vi "JPG_Percentile.vi"(5 "max":u16=97, 7 "min":u16=3, 10 "u16 pixmap 3":T1) -> (2 "unsigned 8bit integer":u8[][](array[numeric]))   [LabVIEW 2020]
uses:
  <vilib>/gmath/NI_Gmath.lvlib
  <vilib>/gmath/statdist.llb/st_Percentiles (scalar).vi
  _controls/img.u16.graph.25pc.axes.ctl
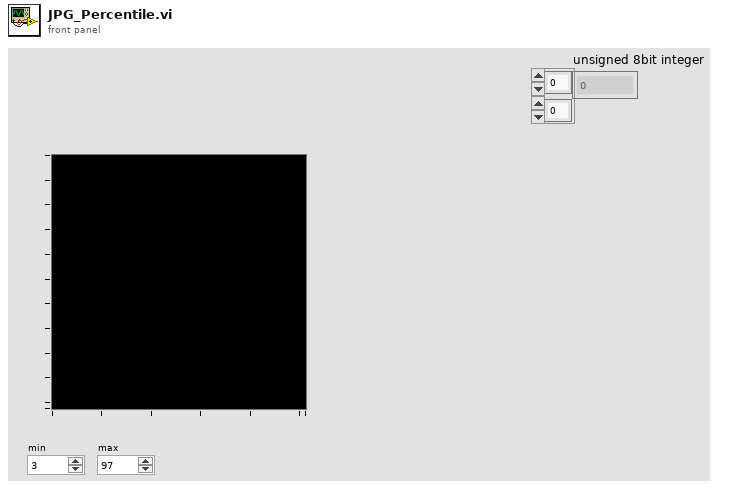
[diagram p1: front panel]
types:
  T1 = typedef "img.u16.graph.25pc.axes.ctl" = u16[][]
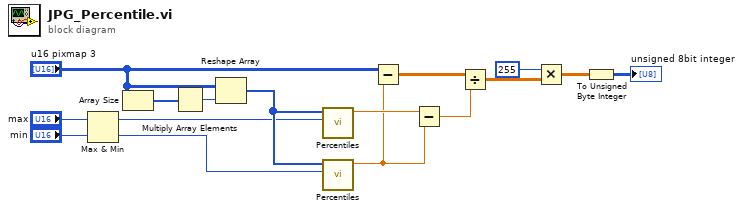
[diagram p0: block diagram]
diagram:
  n1 = Max & Min(x="max", y="min") -> (max(x,y)=w6:u16, min(x,y)=w5:u16)
  n2 = Array Size(array="u16 pixmap 3") -> (size(s)=w13:i32[])
  n3 = Multiply Array Elements(1:w13) -> (0:w12:i32)
  n4 = Reshape Array("u16 pixmap 3", w12) -> (w11:u16[])
  n5 = call-poly <vilib>:"Percentiles.vi"("p"=w6, "x array"=w11) -> ("percentile"=w3:dbl)  [unwired: 8 in, 1 out]
  n6 = call-poly <vilib>:"Percentiles.vi"("p"=w5, "x array"=w11) -> ("percentile"=w2:dbl)  [unwired: 8 in, 1 out]
  n7 = Subtract(x="u16 pixmap 3", y=w2) -> (x-y=w4:dbl[][])
  n8 = Subtract(x=w3, y=w2) -> (x-y=w1:dbl)
  n9 = Divide(x=w4, y=w1) -> (x/y=w16:dbl[][])
  n10 = Multiply(x=u16 255, y=w16) -> (x*y=w14:dbl[][])
  n11 = To Unsigned Byte Integer(number=w14) -> (unsigned 8bit integer=→"unsigned 8bit integer":u8[][])
